vi "CRC16_MAVLink_Checksum_Calculator.vi"(11 "Message":u8[](array[numeric])) -> (1 "Bytes":u8[](array[numeric]) format="%.0x", 2 "Checksum Numeric Hex":u16 format="%.0x")   [LabVIEW 2014]
doc: "MAVLink Checksum Calculator\n\nBrent"
panel:
  # "MAVLink Input  -U  0xFE"
  # "Output"
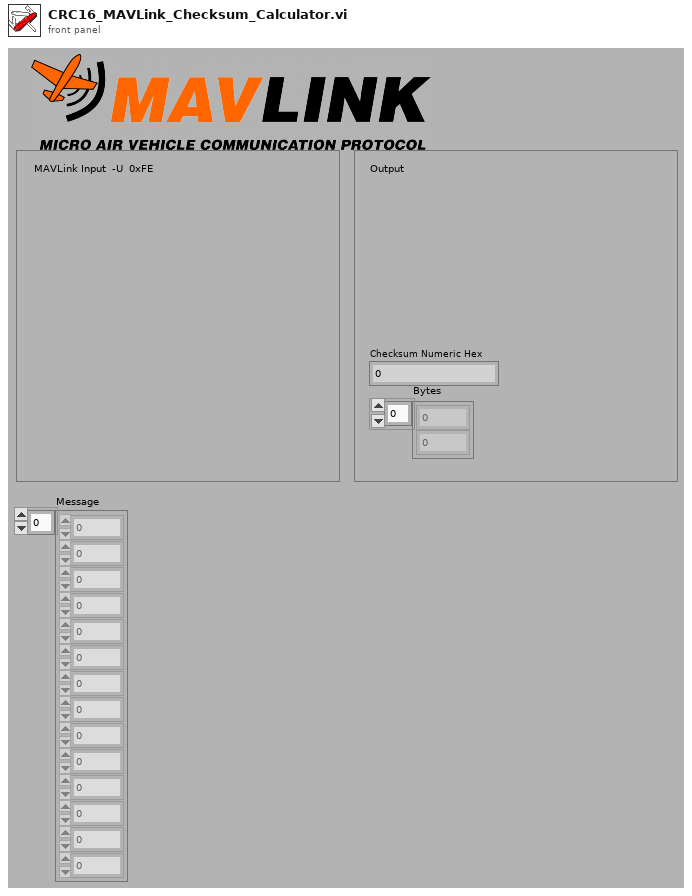
[diagram p1: front panel]
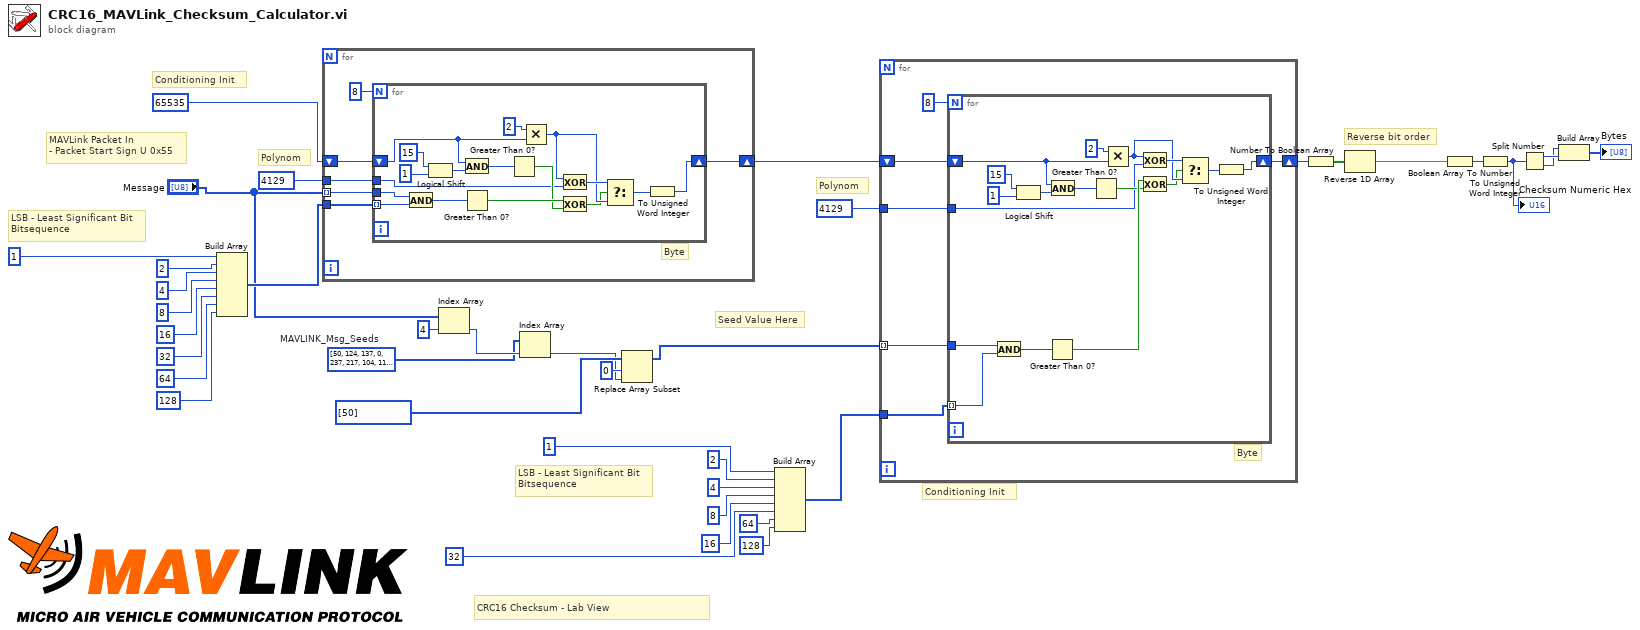
[diagram p0: block diagram]
diagram:
  w6 = u8[] [50, 124, 137, 0, 237, 217, 104, 119, 0, 0, 0, 89, 0, 0, 0, 0, 0, 0, 0, 0, 214, 159, 220, 168, 24, 23, 170, 144, 67, 115, 39, 246, 185, 104, 237, 244, 222, 212, 9, 254, 230, 28, 28, 132, 221, 232, 11, 153, 41, 39, 214, 223, 141, 33, 15, 3, 100, 24, 239, 238, 30, 240, 183, 130, 130, 0, 148, 21, 0, 243, 124, 0, 0, 0, 20, 0, 152, 143, 0, 0, 127, 106, 0, 0, 0, 0, 0, 0, 0, 231, 183, 63, 54, 0, 0, 0, 0, 0, 0, 0, 175, 102, 158, 208, 56, 93, 0, 0, 0, 0, 235, 93, 124, 0, 0, 0, 0, 0, 0, 0, 0, 0, 0, 0, 0, 0, 0, 0, 0, 0, 0, 0, 0, 0, 0, 0, 0, 0, 0, 0, 0, 0, 0, 0, 0, 0, 0, 42, 241, 15, 134, 219, 208, 188, 84, 22, 19, 21, 134, 0, 78, 68, 189, 127, 111, 21, 21, 144, 1, 234, 73, 181, 22, 83, 0, 0, 0, 0, 0, 0, 0, 0, 0, 0, 0, 0, 0, 0, 0, 0, 0, 0, 0, 71, 0, 0, 0, 0, 0, 0, 0, 0, 0, 0, 0, 0, 0, 0, 0, 0, 0, 0, 0, 0, 0, 0, 0, 0, 0, 0, 0, 0, 0, 0, 0, 0, 0, 0, 0, 0, 0, 0, 0, 0, 0, 0, 0, 0, 0, 0, 0, 0, 0, 0, 0, 0, 0, 0, 0, 204, 49, 170, 44, 83, 46, 0]  # MAVLINK_Msg_Seeds
  # "Seed Value Here"
  # "Polynom"
  # "Conditioning Init"
  # "LSB - Least Significant Bit\nBitsequence"
  # "CRC16 Checksum - Lab View"
  # "Reverse bit order"
  # "MAVLink Packet In\n- Packet Start Sign U 0x55"
  # "Polynom"
  # "Conditioning Init"
  # "LSB - Least Significant Bit\nBitsequence"
  n1 = Build Array(u8 1, u8 2, u8 4, u8 8, u8 16, u8 32, u8 64, u8 128) -> (w27:u8[])
  n2 = for {
    shift-right: [w42] -> w10
    shift-left: u16 65535 -> [w44]
    tunnel: "Message" -> [w41] mode=indexing
    tunnel: w27 -> [w40]
    tunnel: u16 4129 -> [w39]
    # "Byte"
    n3 = for {
      N: 8 -> [_]
      shift-right: [w60] -> w42
      shift-left: w44 -> [w50]
      tunnel: w40 -> [w51] mode=indexing
      tunnel: w41 -> [w46]
      tunnel: w39 -> [w45]
      n4 = And(x=w46, y=w51) -> (x .and. y?=w58:u8)
      n5 = Logical Shift(y=u16 15, x=u16 1) -> (x << y=w54:u16)
      n6 = And(x=w50, y=w54) -> (x .and. y?=w53:u16)
      n7 = Greater Than 0?(x=w58) -> (x > 0?=w57:bool)
      n8 = Greater Than 0?(x=w53) -> (x > 0?=w48:bool)
      n9 = Multiply(x=u16 2, y=w50) -> (x*y=w52:u16)
      n10 = Exclusive Or(1:w45, 2:w52) -> (0:w61:u16)
      n11 = Exclusive Or(1:w48, 2:w57) -> (0:w47:bool)
      n12 = Select(t=w61, s=w47, f=w52) -> (s? t:f=w59:u16)
      n13 = To Unsigned Word Integer(number=w59) -> (unsigned 16bit integer=w60:u16)
    }
  }
  n14 = Index Array(array="Message", index=4) -> (element=w7:u8)
  n15 = Index Array(array=w6, index=w7) -> (element=w3:u8)
  n16 = Replace Array Subset(array=u8[] [50] ("unsigned byte array"), new element=w3, index=0) -> (w2:u8[])
  n17 = Build Array(u8 1, u8 2, u8 4, u8 8, u8 16, u8 32, u8 64, u8 128) -> (w19:u8[])
  n18 = for {
    shift-right: [w65] -> w9
    shift-left: w10 -> [w67]
    tunnel: w2 -> [w64] mode=indexing
    tunnel: w19 -> [w63]
    tunnel: u16 4129 -> [w62]
    # "Byte"
    n19 = for {
      N: 8 -> [_]
      shift-right: [w83] -> w65
      shift-left: w67 -> [w73]
      tunnel: w63 -> [w74] mode=indexing
      tunnel: w64 -> [w69]
      tunnel: w62 -> [w68]
      n20 = And(x=w69, y=w74) -> (x .and. y?=w81:u8)
      n21 = Logical Shift(y=u16 15, x=u16 1) -> (x << y=w77:u16)
      n22 = Greater Than 0?(x=w81) -> (x > 0?=w80:bool)
      n23 = And(x=w73, y=w77) -> (x .and. y?=w76:u16)
      n24 = Greater Than 0?(x=w76) -> (x > 0?=w71:bool)
      n25 = Multiply(x=u16 2, y=w73) -> (x*y=w75:u16)
      n26 = Exclusive Or(1:w68, 2:w75) -> (0:w84:u16)
      n27 = Exclusive Or(1:w71, 2:w80) -> (0:w70:bool)
      n28 = Select(t=w84, s=w70, f=w75) -> (s? t:f=w82:u16)
      n29 = To Unsigned Word Integer(number=w82) -> (unsigned 16bit integer=w83:u16)
    }
  }
  n30 = Number To Boolean Array(number=w9) -> (Boolean array=w26:bool[])
  n31 = Reverse 1D Array(array=w26) -> (reversed array=w25:bool[])
  n32 = Boolean Array To Number(Boolean array=w25) -> (number=w24:u32)
  n33 = To Unsigned Word Integer(number=w24) -> (unsigned 16bit integer=w29:u16)
  "Checksum Numeric Hex" <- w29
  n34 = Split Number(x=w29) -> (hi(x)=w22:u8, lo(x)=w21:u8)
  n35 = Build Array(w21, w22) -> (→"Bytes":u8[])
